vi "Auto Angle.vi"(8 "PID Config":T1={"Gains"={"P"=0.1, "I"=0.0, "D"=0.0, "F"=0.0}, "Error Allowed"={"High"=0.0, "Low"=0.0}, "I Zone"={"High"=0.0, "Low"=0.0}, "Peak Out 0-1"={"High"=0.0, "Low"=0.0}, "Max I Accu"={"High"=0.0, "Low"=0.0}} {"Max I Accu"."Low" format="%#.8f"; "Max I Accu"."High" format="%#.8f"; "Gains"."F" format="%#.8f"; "Gains"."D" format="%#.8f"; "Gains"."I" format="%#.8f"; "Gains"."P" format="%#.8f"; "Error Allowed"."Low" format="%#.8f"; "Error Allowed"."High" format="%#.8f"; "I Zone"."Low" format="%#.8f"; "I Zone"."High" format="%#.8f"; "Peak Out 0-1"."Low" format="%#.8f"; "Peak Out 0-1"."High" format="%#.8f"}, 9 "Yaw":T4 scale format="%.3f", 11 "CMD_ACT_SwerveDrive_Data":T6 {"Auto Angle" scale format="%.3f"; "Direction"."Rotate(Yaw) CCW 1 CW -1" scale=1.0..-1.0; "Direction"."Traverse"."Angle" scale format="%.3f"; "Direction"."Traverse"."Velocity" scale=-1.0..1.0 scale format="%.1f"}) -> (1 "At Angle Out":bool, 5 "Mode Out":T7)   [LabVIEW 2023]
uses:
  Shared Code/TypeDefs/Dial_Compase heading unit circle CCW positive.ctl
  Shared Code/TypeDefs/ENUM_Swerve_CMD_Mode Select.ctl
  Shared Code/TypeDefs/Cluster_X-Y.ctl
  Shared Code/TypeDefs/Cluster_High-Low.ctl
  Shared Code/TypeDefs/Cluster_PID Gains.ctl
  Shared Code/TypeDefs/Cluster_SW PID Config.ctl
panel:
  out "CMD_ACT_SwerveDrive_Data 2":T6 {"Auto Angle" scale format="%.3f"; "Direction"."Rotate(Yaw) CCW 1 CW -1" scale=1.0..-1.0; "Direction"."Traverse"."Angle" scale format="%.3f"; "Direction"."Traverse"."Velocity" scale=-1.0..1.0 scale format="%.1f"}
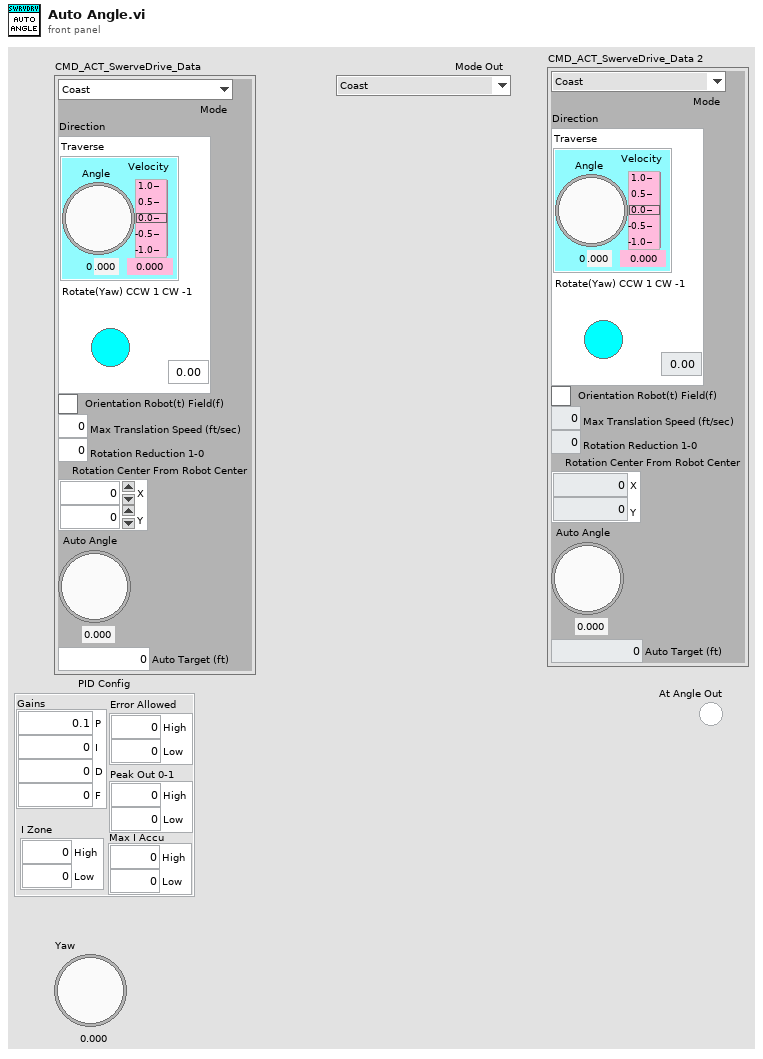
[diagram p1: front panel]
types:
  T1 = typedef "Cluster_SW PID Config.ctl" = cluster{"Gains":T2, "Error Allowed":T3, "I Zone":T3, "Peak Out 0-1":T3, "Max I Accu":T3}
  T2 = typedef "Cluster_PID Gains.ctl" = cluster{"P":dbl, "I":dbl, "D":dbl, "F":dbl}
  T3 = typedef "Cluster_High-Low.ctl" = cluster{"High":dbl, "Low":dbl}
  T4 = typedef "Dial_Compase heading unit circle CCW positive.ctl" = dbl
  T5 = typedef "Cluster_X-Y.ctl" = cluster{"X":dbl, "Y":dbl}
  T6 = cluster{"Mode":enum16{"Coast", "Manual", "Auto Trans Auto Rotate", "Manual Trans Auto Rotate", "Balance", "Stop Brake", "Lock Wheels"}, "Direction":cluster{"Traverse":cluster{"Velocity":dbl, "Angle":T4, "Rotations Count":dbl}, "Rotate(Yaw) CCW 1 CW -1":dbl}, "Orientation Robot(t) Field(f)":bool, "Max Translation Speed (ft/sec)":dbl, "Rotation Reduction 1-0":dbl, "Rotation Center From Robot Center":T5, "Auto Angle":dbl, "Auto Target (ft)":dbl}
  T7 = typedef "ENUM_Swerve_CMD_Mode Select.ctl" = enum16{"Coast", "Manual", "Auto Trans Auto Rotate", "Manual Trans Auto Rotate", "Balance", "Stop Brake", "Lock Wheels"}
  T8 = enum16{"Coast", "Manual", "Auto Trans Auto Rotate", "Manual Trans Auto Rotate", "Balance", "Stop Brake", "Lock Wheels"}
  T9 = typedef "NUM_Rotate Input.ctl" = dbl
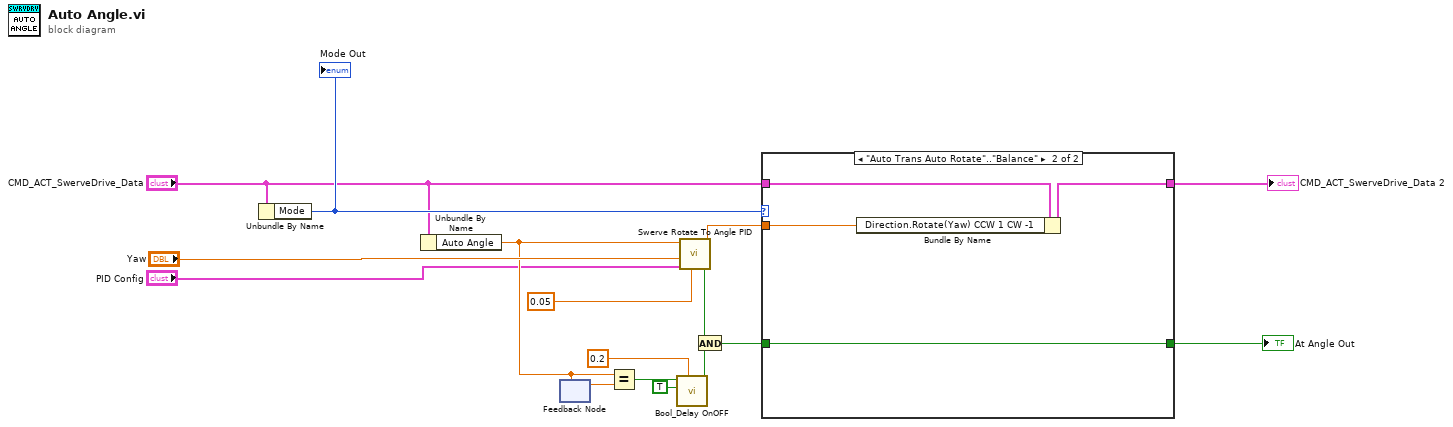
[diagram p0: block diagram]
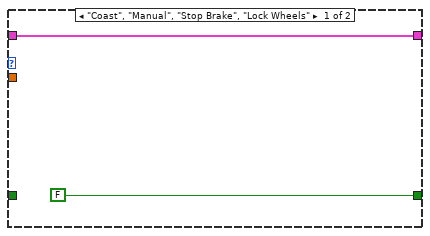
[diagram p2: hidden frame]
diagram:
  n1 = Unbundle By Name("CMD_ACT_SwerveDrive_Data") -> ("Mode"=w15:T8)
  "Mode Out" <- w15
  n2 = Unbundle By Name("CMD_ACT_SwerveDrive_Data") -> ("Auto Angle"=w10:dbl)
  n3 = feedback #1() -> (w11:dbl)  [unwired: 1 in]
  n4 = feedback-in #1(w10) -> ()
  n5 = Equal?(x=w10, y=w11) -> (x = y?=w9:bool)
  n6 = call "Bool_Delay OnOFF.vi"("Delay Time(S)"=0.2, "Delay On(t) Off(f)"=TRUE, "Input"=w9) -> ("Output"=w6:bool)  [unwired: 7 in, 1 out]
  n7 = call "Swerve Rotate To Angle PID.vi"("Target Cycle Time(S)"=0.05, "PID Config"="PID Config", "Current Yaw"="Yaw", "Target Yaw"=w10) -> ("At Angle Out"=w5:bool, "Direction.Rotate(Yaw) CCW 1 CW -1 Out"=w12:T9)  [unwired: 5 in, 1 out]
  n8 = And(x=w5, y=w6) -> (x .and. y?=w4:bool)
  n9 = case shown="\"Auto Trans Auto Rotate\"..\"Balance\"" w15 {
    tunnel: "CMD_ACT_SwerveDrive_Data" -> [w18 w22]
    tunnel: w12 -> [_ w21]
    tunnel: [w18 w20] -> w2
    tunnel: w4 -> [_ w19]
    tunnel: [FALSE w19] -> w3
    frame "Coast", "Manual", "Stop Brake", "Lock Wheels" {
    }
    frame "Auto Trans Auto Rotate".."Balance" {
      n10 = Bundle By Name(cluster=w22, "Direction.Rotate(Yaw) CCW 1 CW -1"=w21) -> (w20:T6)
    }
  }
  "At Angle Out" <- w3
  "CMD_ACT_SwerveDrive_Data 2" <- w2
